vi "GUI Open Login.vi"(8 "error in (no error)":errorcluster, 10 "Password? (F)":bool, 11 "Controller IP Address in":string) -> (0 "error out":errorcluster, 1 "Cancelled?":bool, 2 "Password":string, 3 "Controller IP Address out":string)   [LabVIEW 2011, in "User Interface VIs.lvlib"]
uses:
  User Interface VIs.lvlib
  User Interface Window VIs.lvlib
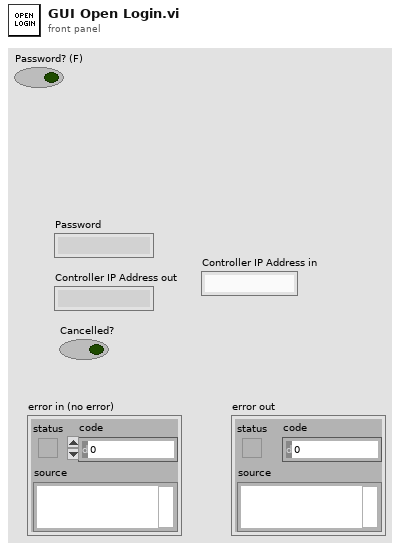
[diagram p1: front panel]
types:
  T1 = enum32{"Invalid", "Standard", "Closed", "Hidden", "Minimized", "Maximized"}
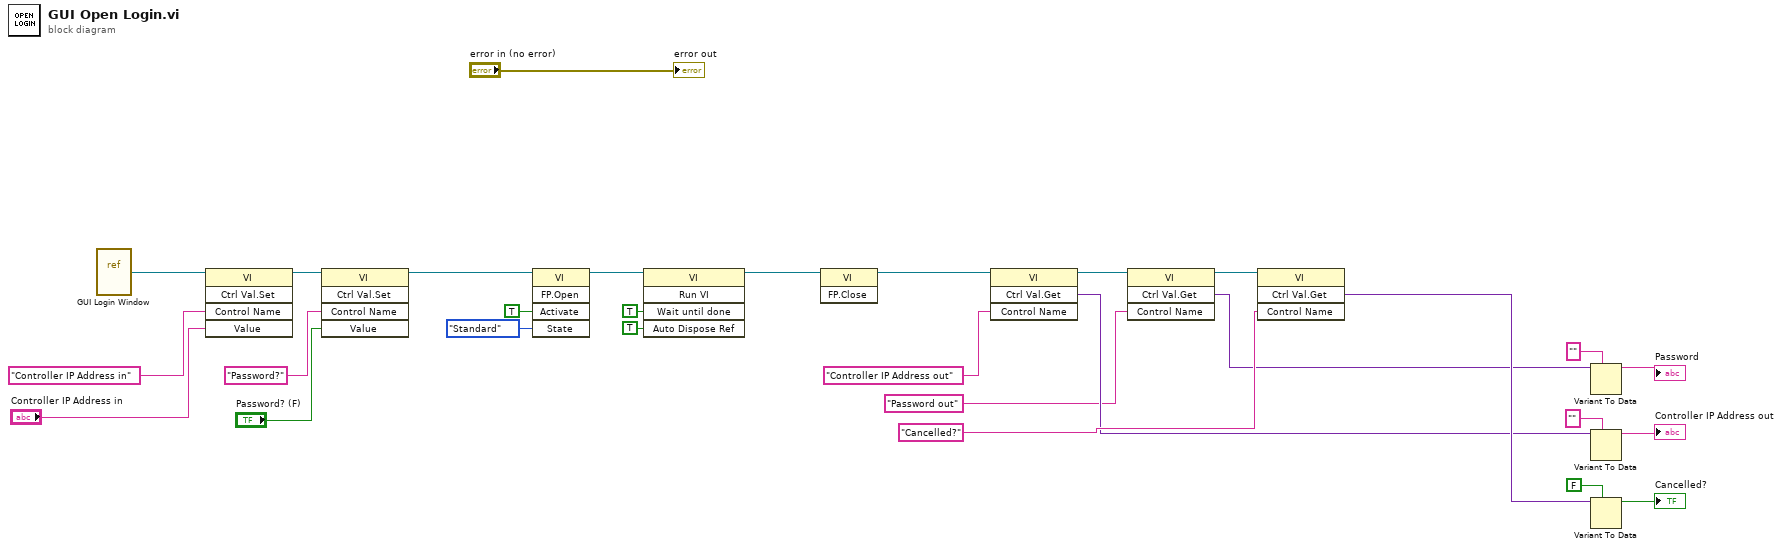
[diagram p0: block diagram]
diagram:
  n1 = vi-ref "GUI Login Window.vi"() -> (w29:refnum<vi>)
  n2 = invoke class="VI" method="Ctrl Val.Set"(reference=w29, "Control Name"="Controller IP Address in", "Value"="Controller IP Address in") -> (reference out=w4:refnum<vi>)  [unwired: 2 in, 4 out]
  n3 = invoke class="VI" method="Ctrl Val.Set"(reference=w4, "Control Name"="Password?", "Value"="Password? (F)") -> (reference out=w3:refnum<vi>)  [unwired: 2 in, 4 out]
  n4 = invoke class="VI" method="FP.Open"(reference=w3, "Activate"=TRUE ("Activate?"), "State"=T1."Standard") -> (reference out=w8:refnum<vi>)  [unwired: 2 in, 4 out]
  n5 = invoke class="VI" method="Run VI"(reference=w8, "Wait until done"=TRUE ("Wait Until Done"), "Auto Dispose Ref"=TRUE ("Auto Dispose Reference")) -> (reference out=w7:refnum<vi>)  [unwired: 2 in, 4 out]
  n6 = invoke class="VI" method="FP.Close"(reference=w7) -> (reference out=w6:refnum<vi>)  [unwired: 2 in, 2 out]
  n7 = invoke class="VI" method="Ctrl Val.Get"(reference=w6, "Control Name"="Controller IP Address out") -> (reference out=w15:refnum<vi>, "Get Control Value Variant"=w18:variant)  [unwired: 2 in, 2 out]
  n8 = invoke class="VI" method="Ctrl Val.Get"(reference=w15, "Control Name"="Password out") -> (reference out=w23:refnum<vi>, "Get Control Value Variant"=w19:variant)  [unwired: 2 in, 2 out]
  n9 = invoke class="VI" method="Ctrl Val.Get"(reference=w23, "Control Name"="Cancelled?") -> ("Get Control Value Variant"=w27:variant)  [unwired: 2 in, 3 out]
  n10 = Variant To Data(type="" ("Control Name"), Variant=w19) -> (data=→"Password":string)  [unwired: 1 in, 1 out]
  n11 = Variant To Data(type="" ("Control Name"), Variant=w18) -> (data=→"Controller IP Address out":string)  [unwired: 1 in, 1 out]
  n12 = Variant To Data(type=FALSE ("Stop?"), Variant=w27) -> (data=→"Cancelled?":bool)  [unwired: 1 in, 1 out]
  "error out" <- "error in (no error)"
